vi "P_Trig.vi"(11 "In":bool) -> (3 "Q":bool)   [LabVIEW 2020]
panel:
  out "Memory bit":bool
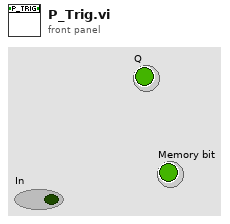
[diagram p1: front panel]
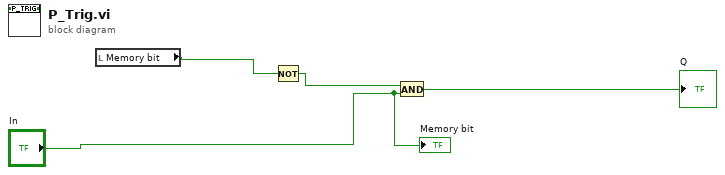
[diagram p0: block diagram]
diagram:
  n1 = local read "Memory bit"() -> (w1:bool)
  n2 = Not(x=w1) -> (.not. x?=w4:bool)
  n3 = And(x=w4, y="In") -> (x .and. y?=→"Q":bool)
  "Memory bit" <- "In"
